vi "PQsetClientEncoding.vi"(8 "error in (no error)":errorcluster, 10 "encoding":string, 11 "conn":u64) -> (0 "error out":errorcluster, 2 "PQsetClientEncoding":i64)   [LabVIEW 2019, in "libpqlv64.lvlib"]
uses:
  libpqlv64.lvlib
  libpq.dll
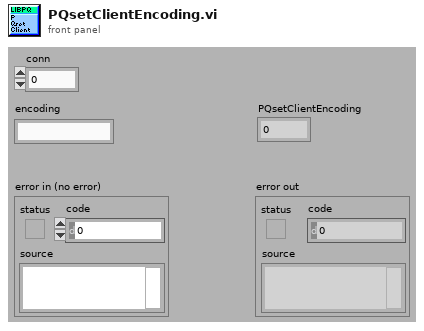
[diagram p1: front panel]
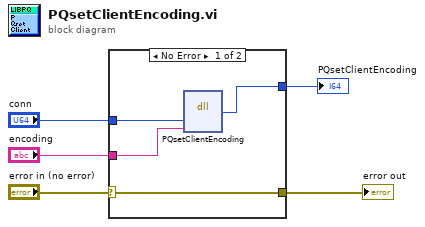
[diagram p0: block diagram]
diagram:
  n1 = case shown="No Error" "error in (no error)" {
    selector: "error in (no error)" -> [w9 w10]
    tunnel: [w9 w10] -> w4
    tunnel: [w8 _] -> w3
    tunnel: "encoding" -> [w7 _]
    tunnel: "conn" -> [w6 _]
    frame No Error {
      n2 = dll-call lib="libpq.*" fn="PQsetClientEncoding"("conn"=w6, "encoding"=w7) -> ("PQsetClientEncoding"=w8:i64)  [unwired: 5 in, 2 out]
    }
    frame Error {
    }
  }
  "PQsetClientEncoding" <- w3
  "error out" <- w4
